vi "Read Run Time Configuration.vi"(8 "error in (no error)":errorcluster, 11 "Session in":refnum<class "Plugin Session.lvclass">) -> (0 "error out":errorcluster, 2 "Run Time Configuration":string, 3 "Session out":refnum<class "Plugin Session.lvclass">)   [LabVIEW 2023, in "InstrumentStudio Plugin SDK.lvlib" / "Plugin Session.lvclass"]
doc: "Call this VI to read the run-time configuration string for your plugin panel."
uses:
  Plugin Session.lvclass
  Plugin Session.lvclass/Plugin Session.ctl
  Read Session Id.vi
  NationalInstruments.VIHost.Interop.dll
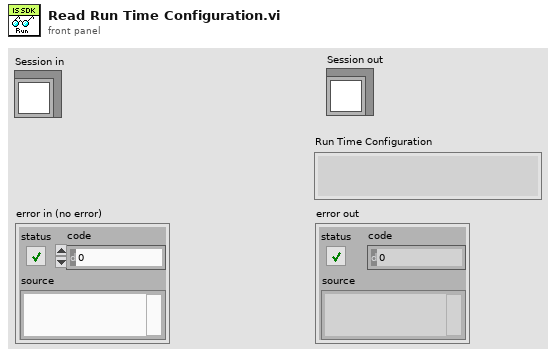
[diagram p1: front panel]
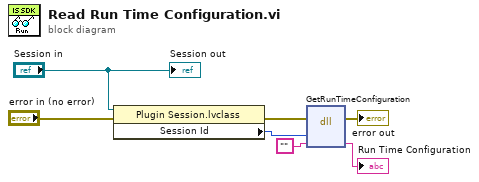
[diagram p0: block diagram]
diagram:
  n1 = property class="Plugin Session.lvclass"(reference="Session in", error in="error in (no error)") -> (error out=w5:errorcluster, "Session Id"=w2:u64)  [unwired: 1 out]
  n2 = dll-call lib="C:/Users/nmurphy/Downloads/InstrumentStudio_LabVIEW_Plugins/LabVIEW/ExampleProject/PluginSDK/NationalInstruments.VIHost.Interop.dll" fn="GetRunTimeConfiguration"(error in=w5, "hostId"=w2, "configuration"="") -> (error out=→"error out":errorcluster, "configuration"=→"Run Time Configuration":string)  [unwired: 4 in, 1 out]
  "Session out" <- "Session in"
